vi "Send Response.vi"(8 "error in (no error)":errorcluster, 9 "timeout in ms (0)":i32 format="%d ms", 10 "response":T1, 11 "Dispatcher in":refnum<class "Dispatcher Thread.lvclass">) -> (0 "error out":errorcluster, 3 "Dispatcher out":refnum<class "Dispatcher Thread.lvclass">)   [LabVIEW 2017, in "DSF Core.lvlib" / "Dispatcher Thread.lvclass"]
uses:
  Dispatcher Thread.lvclass
  Interface/Dispatcher/Response Data.ctl
  Interface/Dispatcher/Response.ctl
  Interface/Dispatcher/Parameters.ctl
  Dispatcher Thread.lvclass/Dispatcher Thread.ctl
  Interface/Dispatcher/Write Dispatcher Response.vi
  Interface/Dispatcher/Dispatcher Interface.lvclass
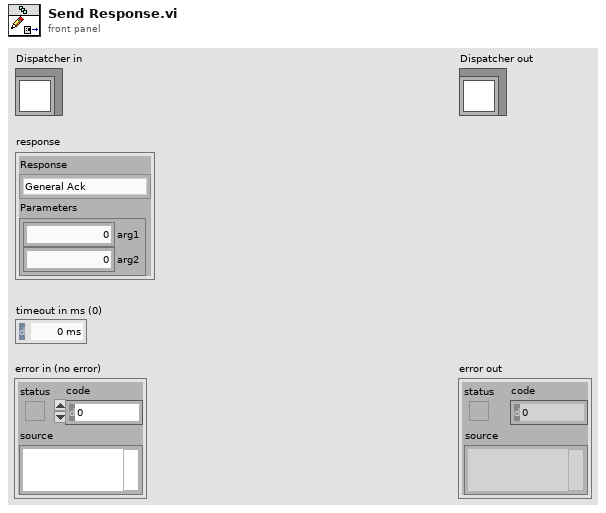
[diagram p1: front panel]
types:
  T1 = typedef "DSF Core.lvlib/Dispatcher Interface.lvclass/Response Data.ctl" = cluster{"Response":T2, "Parameters":T3}
  T2 = typedef "DSF Core.lvlib/Dispatcher Interface.lvclass/Response.ctl" = enum8{"General Ack", "Error", "Shutting Down"}
  T3 = typedef "DSF Core.lvlib/Dispatcher Interface.lvclass/Parameters.ctl" = cluster{"arg1":u64, "arg2":u64}
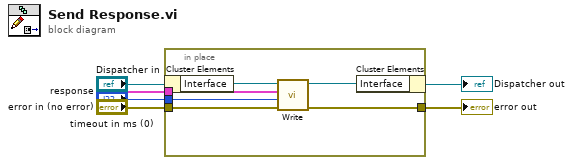
[diagram p0: block diagram]
diagram:
  n1 = in-place {
    in-place-border: "error in (no error)" -> [w10]
    in-place-border: [w9] -> w4
    in-place-border: "timeout in ms (0)" -> [w8]
    in-place-border: "response" -> [w7]
    n2 = in-place-cluster #1("Dispatcher in") -> ("Interface"=w12:refnum<class "Dispatcher Interface.lvclass">)
    n3 = call-poly "Write.vi"("error in (no error)"=w10, "timeout in ms (0)"=w8, "response"=w7, "Dispatcher Interface in"=w12) -> ("error out"=w9:errorcluster, "Dispatcher Interface out"=w11:refnum<class "Dispatcher Interface.lvclass">)  [unwired: 6 in]
    n4 = in-place-cluster #1("Interface"=w11) -> (→"Dispatcher out":refnum<class "Dispatcher Thread.lvclass">)
  }
  "error out" <- w4
